vi "MerweScSigPts_SigmaPoints.vi"(9 "P":T1, 10 "X":T1, 11 "MerweScaledSigmaPts":T2) -> (0 "Error":bool, 3 "SigmaPoints":T1)   [LabVIEW 2019, in "Trajectory_Library.lvlib"]
doc: "Computes the sigma points for an unscented Kalman filter given the mean (x) and covariance(P)\nof the filter.\n \nInputs:\n - MerweScaledSigmaPts -- data cluster\n - x -- An array of the means.\n - P -- Covariance of the filter.\n\nOutputs:\n - SigmaPoints -- Two dimensional array of sigma points. Each column contains all of the sigmas for one dimension in the problem space. Ordered by Xi_0, Xi_{1..n}, Xi_{n+1..2n}.\n - Error -- If TRUE, an error occured."
uses:
  Trajectory_Library.lvlib
  MERWE_SCALED_SIGMA_PTS.ctl
  <vilib>/Analysis/Matrix/Datatypes/RealMatrix.ctl
  <vilib>/Analysis/Matrix/Numeric/Multiply/Multiply - RM,R.vi
  <vilib>/Analysis/Matrix/Numeric/Subtract/Subtract - RM,RM.vi
  <vilib>/Analysis/Matrix/Numeric/Add/Add - RM,RM.vi
  <vilib>/Analysis/Matrix/NI_Matrix.lvlib
panel:
  # "<?, 1>"
  # "<?, 1>"
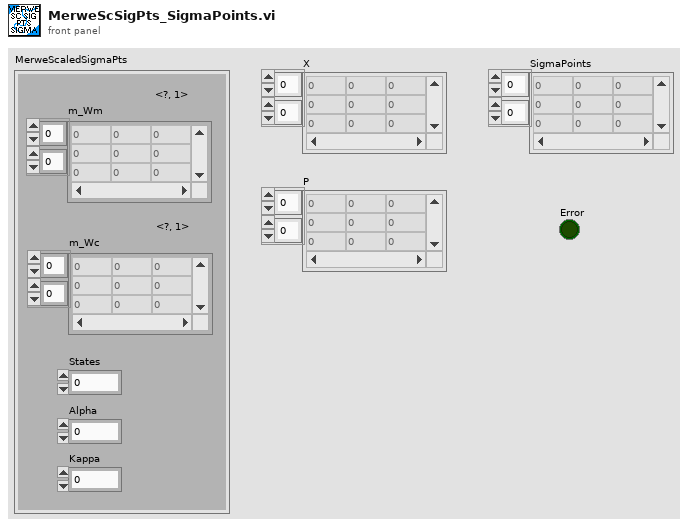
[diagram p1: front panel]
types:
  T1 = typedef "NI_Matrix.lvlib/RealMatrix.ctl" = dbl[][]
  T2 = typedef "Trajectory_Library.lvlib/MERWE_SCALED_SIGMA_PTS.ctl" = cluster{"m_Wm":T1, "States":i32, "Alpha":dbl, "m_Wc":T1, "Kappa":i32}
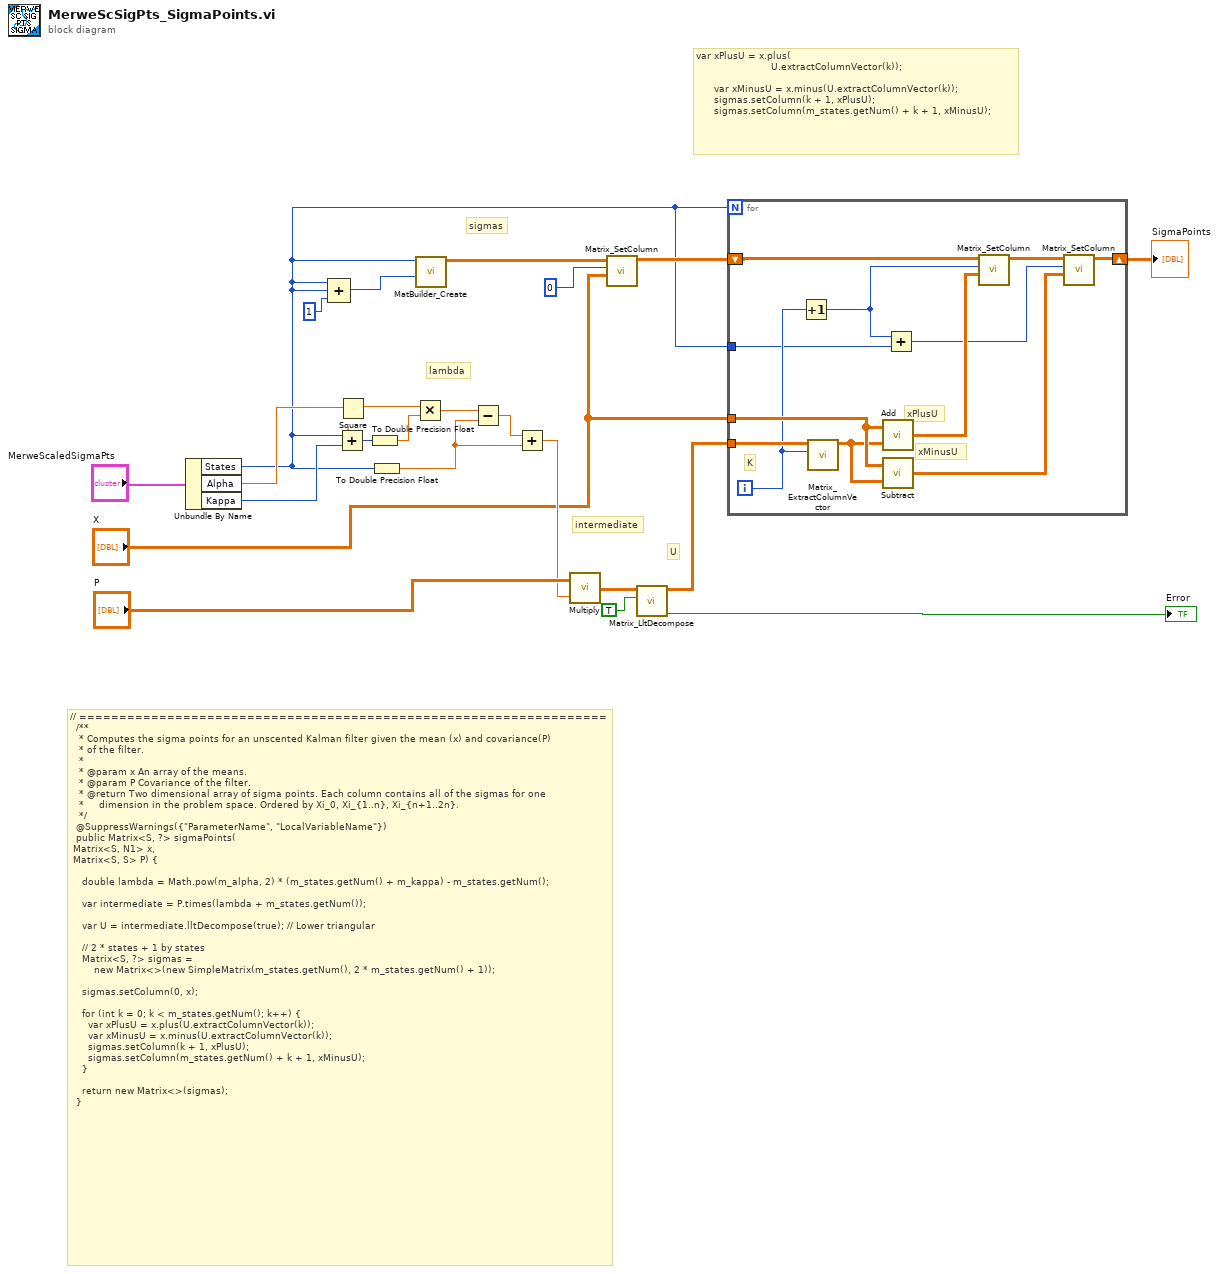
[diagram p0: block diagram]
diagram:
  # "U"
  # "var xPlusU = x.plus(\n                         U.extractColumnVector(k));\n\n      var xMinusU = x.minus(U.extractColumnVector(k));\n      sigmas.setColumn(k + 1, xPlusU);\n      sigmas.setColumn(m_states.getNum() + k + 1, xMinusU);"
  # "sigmas"
  # "intermediate"
  # "lambda"
  # "// ==================================================================\n  /**\n   * Computes the sigma points for an unscented Kalman filter given the mean (x) and covariance(P)\n   * of the filter.\n   *\n   * @param x An array of the means.\n   * @param P Covariance of the filter.\n   * @return Two dimensional array of sigma points. Each column contains all of the sigmas for one\n   *     dimension in the problem space. Ordered by Xi_0, Xi_{1..n}, Xi_{n+1..2n}.\n   */\n  @SuppressWarnings({\"ParameterName\", \"LocalVariableName\"})\n  public Matrix<S, ?> sigmaPoints(\n\tMatrix<S, N1> x, \n\tMatrix<S, S> P) {\n\n    double lambda = Math.pow(m_alpha, 2) * (m_states.getNum() + m_kappa) - m_states.getNum();\n\n    var intermediate = P.times(lambda + m_states.getNum());\n\n    var U = intermediate.lltDecompose(true); // Lower triangular\n\n    // 2 * states + 1 by states\n    Matrix<S, ?> sigmas =\n        new Matrix<>(new SimpleMatrix(m_states.getNum(), 2 * m_states.getNum() + 1));\n\n    sigmas.setColumn(0, x);\n\n    for (int k = 0; k < m_states.getNum(); k++) {\n      var xPlusU = x.plus(U.extractColumnVector(k));\n      var xMinusU = x.minus(U.extractColumnVector(k));\n      sigmas.setColumn(k + 1, xPlusU);\n      sigmas.setColumn(m_states.getNum() + k + 1, xMinusU);\n    }\n\n    return new Matrix<>(sigmas);\n  }"
  n1 = Unbundle By Name("MerweScaledSigmaPts") -> ("States"=w5:i32, "Alpha"=w18:dbl, "Kappa"=w17:i32)
  n2 = Compound Arithmetic op=ADD(w5, w5, 1 ("value")) -> (w11:i32)
  n3 = Add(x=w5, y=w17) -> (x+y=w22:i32)
  n4 = Square(x=w18) -> (x^2=w19:dbl)
  n5 = To Double Precision Float(number=w22) -> (double precision float=w21:dbl)
  n6 = To Double Precision Float(number=w5) -> (double precision float=w15:dbl)
  n7 = Multiply(x=w19, y=w21) -> (x*y=w20:dbl)
  n8 = call "MatBuilder_Create.vi"("Columns"=w11, "Rows"=w5) -> ("output matrix"=w10:T1)  [unwired: 9 in]
  n9 = Subtract(x=w20, y=w15) -> (x-y=w16:dbl)
  n10 = Add(x=w16, y=w15) -> (x+y=w13:dbl)
  n11 = call-poly <vilib>:"Multiply.vi"("Real Scalar c"=w13, "Real Matrix A"="P") -> ("A * c"=w4:T1)
  n12 = call "Matrix_SetColumn.vi"("Fill Vector"="X", "Column"=0, "input matrix"=w10) -> ("output matrix"=w7:T1)  [unwired: 7 in, 1 out]
  n13 = call "Matrix_LltDecompose.vi"("LowerTriangle"=TRUE, "input matrix"=w4) -> ("Error"=→"Error":bool, "output Cholesky Decomp"=w3:T1)  [unwired: 8 in]
  n14 = for {
    N: w5 -> [_]
    tunnel: w3 -> [w35]
    tunnel: "X" -> [w34]
    shift-right: [w30] -> w6
    shift-left: w7 -> [w32]
    tunnel: w5 -> [w25]
    i -> [w27]
    # "xMinusU"
    # "xPlusU"
    # "K"
    n15 = Increment(x=w27) -> (x+1=w26:i32)
    n16 = call "Matrix_ExtractColumnVector.vi"("Column"=w27, "input matrix"=w35) -> ("output column"=w33:T1)  [unwired: 8 in, 1 out]
    n17 = call-poly <vilib>:"Add.vi"("Real Matrix B"=w33, "Real Matrix A"=w34) -> ("A + B"=w28:T1)
    n18 = call-poly <vilib>:"Subtract.vi"("Real Matrix B"=w33, "Real Matrix A"=w34) -> ("A - B"=w29:T1)
    n19 = Add(x=w26, y=w25) -> (x+y=w24:i32)
    n20 = call "Matrix_SetColumn.vi"("Fill Vector"=w28, "Column"=w26, "input matrix"=w32) -> ("output matrix"=w31:T1)  [unwired: 7 in, 1 out]
    n21 = call "Matrix_SetColumn.vi"("Fill Vector"=w29, "Column"=w24, "input matrix"=w31) -> ("output matrix"=w30:T1)  [unwired: 7 in, 1 out]
  }
  "SigmaPoints" <- w6
